vi "move picture core.vi"(0 "data string in":string, 1 "picture op-code":T1 items=["set pixel"=4, "move pen"=5, "move pen to"=6, "draw line"=7, "draw line to"=8, "rectangle frame"=9, "rectangle fill"=10, "oval frame"=11, "oval fill"=12, "arc frame"=13, "arc fill"=14, "gray out rect"=15, "poly line"=16, "poly line fill"=17, "text box"=18, "round rect frame"=24, "round rect fill"=25, "copy pixmap"=29, "new font"=0, "copy pixmap with mask"=40, "select pen"=41], 3 "move":cluster{"y":i16, "x":i16}) -> (14 "data string out":string)   [LabVIEW 2019]
uses:
  picture op-code.ctl
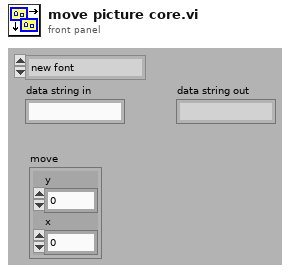
[diagram p1: front panel]
types:
  T1 = typedef "picture op-code.ctl" = u16
  T2 = cluster{"top":i16, "left":i16, "bottom":i16, "right":i16}
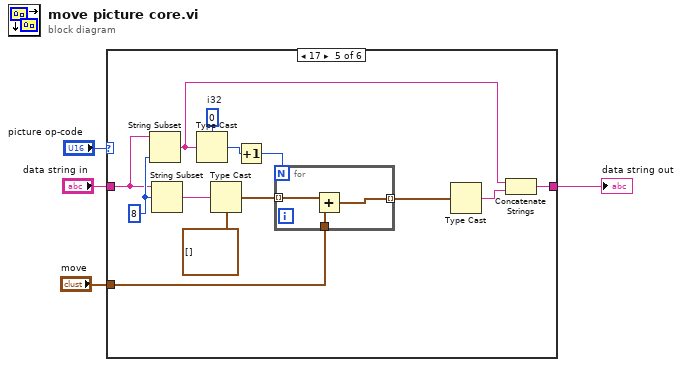
[diagram p0: block diagram]
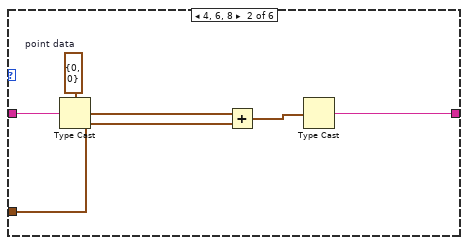
[diagram p3: hidden frame]
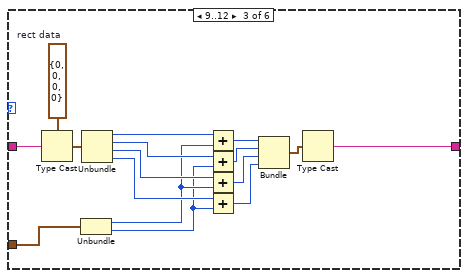
[diagram p4: hidden frame]
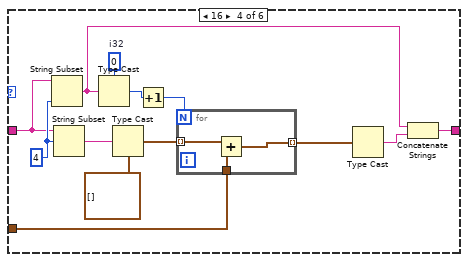
[diagram p5: hidden frame]
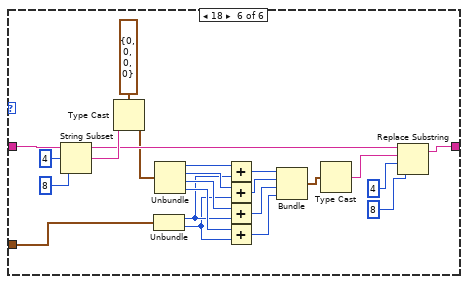
[diagram p6: hidden frame]
diagram:
  n1 = case shown="17" "picture op-code" {
    tunnel: "data string in" -> [w5 w11 w27 w37 w53 w79]
    tunnel: [w5 w10 w26 w34 w50 w61] -> w3
    tunnel: "move" -> [_ w9 w19 w33 w49 w62]
    frame Default {
    }
    frame 4, 6, 8 {
      w8 = cluster{"y":i16, "x":i16} {"y"=0, "x"=0}  # point data
      n2 = Type Cast(type=w8, x=w11) -> (*(type *) &x=w7:cluster{"y":i16, "x":i16})
      n3 = Add(x=w7, y=w9) -> (x+y=w6:cluster{"y":i16, "x":i16})
      n4 = Type Cast(x=w6) -> (*(type *) &x=w10:string)  [unwired: 1 in]
    }
    frame 9..12 {
      w25 = T2 {"top"=0, "left"=0, "bottom"=0, "right"=0}  # rect data
      n5 = Type Cast(type=w25, x=w27) -> (*(type *) &x=w24:T2)
      n6 = Unbundle(w19) -> ("y"=w18:i16, "x"=w17:i16)
      n7 = Unbundle(w24) -> ("top"=w23:i16, "left"=w21:i16, "bottom"=w22:i16, "right"=w20:i16)
      n8 = Add(x=w23, y=w18) -> (x+y=w16:i16)
      n9 = Add(x=w21, y=w17) -> (x+y=w15:i16)
      n10 = Add(x=w22, y=w18) -> (x+y=w14:i16)
      n11 = Add(x=w20, y=w17) -> (x+y=w13:i16)
      n12 = Bundle(w16, w15, w14, w13) -> (w12:cluster{i16, i16, i16, i16})  [unwired: 1 in]
      n13 = Type Cast(x=w12) -> (*(type *) &x=w26:string)  [unwired: 1 in]
    }
    frame 16 {
      w40 = 0  # i32
      w38 = 4 ("length (rest)")
      n14 = String Subset(string=w37, length (rest)=w38) -> (substring=w35:string)  [unwired: 1 in]
      n15 = String Subset(string=w37, offset (0)=w38) -> (substring=w31:string)  [unwired: 1 in]
      n16 = Type Cast(type=w40, x=w35) -> (*(type *) &x=w29:i32)
      n17 = Type Cast(type=cluster{"y":i16, "x":i16}[] [], x=w31) -> (*(type *) &x=w36:cluster{"y":i16, "x":i16}[])
      n18 = Increment(x=w29) -> (x+1=w28:i32)
      n19 = for {
        N: w28 -> [_]
        tunnel: w36 -> [w42] mode=indexing
        tunnel: [w41] -> w39 mode=indexing
        tunnel: w33 -> [w43]
        n20 = Add(x=w42, y=w43) -> (x+y=w41:cluster{"y":i16, "x":i16})
      }
      n21 = Type Cast(x=w39) -> (*(type *) &x=w30:string)  [unwired: 1 in]
      n22 = Concatenate Strings(w35, w30) -> (w34:string)
    }
    frame 17 {
      w56 = 0  # i32
      w54 = 8 ("length (rest)")
      n23 = String Subset(string=w53, length (rest)=w54) -> (substring=w51:string)  [unwired: 1 in]
      n24 = String Subset(string=w53, offset (0)=w54) -> (substring=w47:string)  [unwired: 1 in]
      n25 = Type Cast(type=w56, x=w51) -> (*(type *) &x=w45:i32)
      n26 = Type Cast(type=cluster{"y":i16, "x":i16}[] [], x=w47) -> (*(type *) &x=w52:cluster{"y":i16, "x":i16}[])
      n27 = Increment(x=w45) -> (x+1=w44:i32)
      n28 = for {
        N: w44 -> [_]
        tunnel: w52 -> [w58] mode=indexing
        tunnel: [w57] -> w55 mode=indexing
        tunnel: w49 -> [w59]
        n29 = Add(x=w58, y=w59) -> (x+y=w57:cluster{"y":i16, "x":i16})
      }
      n30 = Type Cast(x=w55) -> (*(type *) &x=w46:string)  [unwired: 1 in]
      n31 = Concatenate Strings(w51, w46) -> (w50:string)
    }
    frame 18 {
      n32 = String Subset(string=w79, offset (0)=4, length (rest)=8 ("length (rest)")) -> (substring=w81:string)
      n33 = Type Cast(type=T2 {"top"=0, "left"=0, "bottom"=0, "right"=0} ("output cluster"), x=w81) -> (*(type *) &x=w63:T2)
      n34 = Unbundle(w62) -> ("y"=w70:i16, "x"=w69:i16)
      n35 = Unbundle(w63) -> ("top"=w74:i16, "left"=w72:i16, "bottom"=w73:i16, "right"=w71:i16)
      n36 = Add(x=w74, y=w70) -> (x+y=w68:i16)
      n37 = Add(x=w72, y=w69) -> (x+y=w67:i16)
      n38 = Add(x=w73, y=w70) -> (x+y=w66:i16)
      n39 = Add(x=w71, y=w69) -> (x+y=w65:i16)
      n40 = Bundle(w68, w67, w66, w65) -> (w64:cluster{i16, i16, i16, i16})  [unwired: 1 in]
      n41 = Type Cast(x=w64) -> (*(type *) &x=w60:string)  [unwired: 1 in]
      n42 = Replace Substring(2:8 ("length (rest)"), 3:4 ("offset (0)"), 4:w60, 5:w79) -> (1:w61:string)  [unwired: 1 out]
    }
  }
  "data string out" <- w3
